vi "ctype.vi"(9 "Content-Type":string) -> (1 "ctype":string)   [LabVIEW 2020]
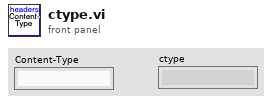
[diagram p1: front panel]
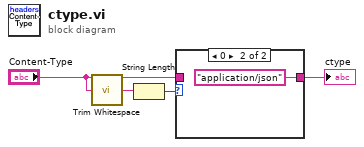
[diagram p0: block diagram]
diagram:
  n1 = call <vilib>:"Trim Whitespace.vi"("string"="Content-Type") -> ("trimmed string"=w1:string)  [unwired: 1 in]
  n2 = String Length(string=w1) -> (length=w3:i32)
  n3 = case shown="0" w3 {
    tunnel: [w5 "application/json"] -> w4
    tunnel: "Content-Type" -> [w5 _]
    frame Default {
    }
    frame 0 {
    }
  }
  "ctype" <- w4
